vi "LNA Return Message.vi"(8 "Error In":errorcluster, 10 "LNA Return Message Msg":refnum<class "LNA Return Message Msg.lvclass">, 11 "TestLNA in":refnum<class "TestLNA.lvclass">) -> (0 "Error Out":errorcluster, 3 "TestLNA out":refnum<class "TestLNA.lvclass">)   [LabVIEW 2016, in "TestLNA.lvlib" / "TestLNA.lvclass"]
doc: "Display dialog with info about returned message."
uses:
  TestLNA.lvclass
  C:/User/Brand/LVP/CSPP-Dev/Packages/CSPP_Core/Actors/CS++BaseActor/CS++BaseActor.lvclass
  LNA Messages/LNA Return Message Msg/LNA Return Message Msg.lvclass
  C:/Program Files (x86)/National Instruments/LabVIEW 2016/vi.lib/NI/Actors/Linked Network Actor/Linked Network Actor Messages/LNA Return Message Msg/LNA Return Message Msg.lvclass
  CSPP_Core/Actors/CS++BaseActor/CS++BaseActor.lvclass/CS++BaseActor.ctl
  CSPP_Core/Actors/CS++BaseActor/Read Object Name.vi
  <vilib>/NI/Actors/Linked Network Actor/Linked Network Actor Messages/LNA Return Message Msg/LNA Return Message Msg.lvclass
  CSPP_Core/Libraries/Utilities/CS++Utilities.lvlib
  <vilib>/ActorFramework/Message/Message.lvclass
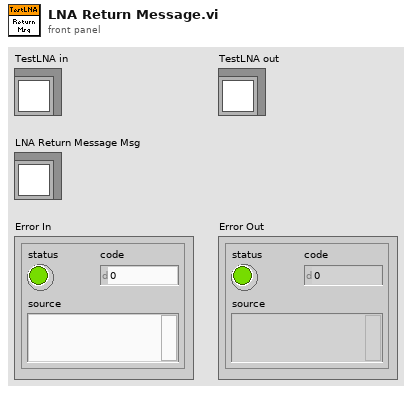
[diagram p1: front panel]
types:
  T1 = typedef "Actor Framework.lvlib/Message Enqueuer.lvclass/Message Priority.ctl" = enum16{"Low", "Normal", "High"}
  T2 = cluster{"Tx Message":refnum<class "Message.lvclass">, "Tx Error":errorcluster, "Message Priority":T1}
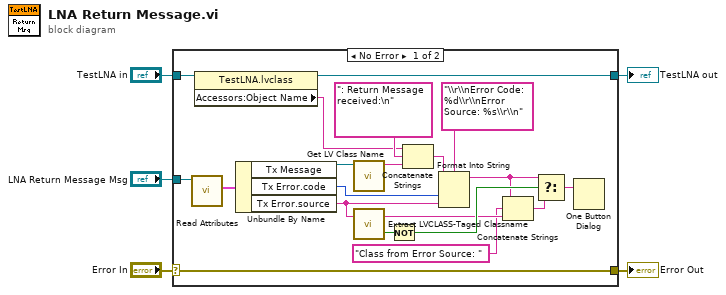
[diagram p0: block diagram]
diagram:
  n1 = case shown="No Error" "Error In" {
    selector: "Error In" -> [w24 w27]
    tunnel: [w24 w27] -> w4
    tunnel: [w15 w26] -> w2
    tunnel: "TestLNA in" -> [w25 w26]
    tunnel: "LNA Return Message Msg" -> [w17 _]
    frame No Error {
      n2 = call <vilib>:"Read Attributes.vi"("Abstract Message Template in"=w17) -> ("Payload"=w23:T2)  [unwired: 9 in, 1 out]
      n3 = property class="TestLNA.lvclass"(reference=w25) -> (reference out=w15:refnum<class "TestLNA.lvclass">, "Accessors:Object Name"=w14:string)  [unwired: 1 in, 1 out]
      n4 = Unbundle By Name(w23) -> ("Tx Message"=w22:refnum<class "Message.lvclass">, "Tx Error.code"=w19:i32, "Tx Error.source"=w13:string)
      n5 = call <vilib>:"Get LV Class Name.vi"("object"=w22) -> ("class name"=w21:string)  [unwired: 9 in, 1 out]
      n6 = call "Extract LVCLASS-Taged Classname.vi"("Tagged LVClass Name"=w13) -> ("found?"=w12:bool, "LVClass Name"=w9:string)
      n7 = Not(x=w12) -> (.not. x?=w11:bool)
      n8 = Concatenate Strings(w14, ": Return Message received:\n", w21) -> (w20:string)
      n9 = Format Into String(format string="\\r\\nError Code: %d\\r\\nError Source: %s\\r\\n", initial string=w20, w19, w13) -> (resulting string=w7:string)  [unwired: 1 in, 1 out]
      n10 = Concatenate Strings(w7, "Class from Error Source: " ("format string"), w9) -> (w8:string)
      n11 = Select(t=w7, s=w11, f=w8) -> (s? t:f=w10:string)
      n12 = One Button Dialog(message=w10) -> ()  [unwired: 1 in, 1 out]
    }
    frame Error {
    }
  }
  "Error Out" <- w4
  "TestLNA out" <- w2
